vi "Data Access Client.vi"() -> ()   [LabVIEW 2019, in "OPC UA Demo.lvlib"]
doc: "Demonstrates the use of the <B>OPC UA Data Access Client VIs</B> to programmatically create an OPC UA client and connects the OPC UA client to an OPC UA server."
uses:
  OPC UA Demo.lvlib
  <vilib>/OPCUA/controls/NodeIds.ctl
  <vilib>/OPCUA/controls/NodeId.ctl
  <vilib>/OPCUA/controls/Write Variant Request.ctl
  <vilib>/OPCUA/controls/Write Status.ctl
  <vilib>/OPCUA/client/Multiple Write Variant.vi
  <vilib>/OPCUA/NI OPC UA Client.lvlib
panel:
  out "data 2":bool
  in  "stop 2":bool
  in  "security policy":T1={"message mode"=enum."Sign", "security"=enum."Basic256"}
  in  "Device.Node.Set Point":i32=1000
  out "Waveform Chart":i32(graph)
  in  "stop":bool
  in  "server endpoint URL":string="opc.tcp://localhost:49580"
  # "Overview: Demonstrates the use of the OPC UA Data Access Client VIs to programmatically create an OPC UA client and connect \nthe OPC UA client to an OPC UA server.\nRequirements: \n1. LabVIEW OPC UA Toolkit\n2. Run this VI on RT targets or Windows\nInstructions:\n1. Specify the server endpoint URL generated by the server.\n2. Specify the security policy.\n3. Run the VI."
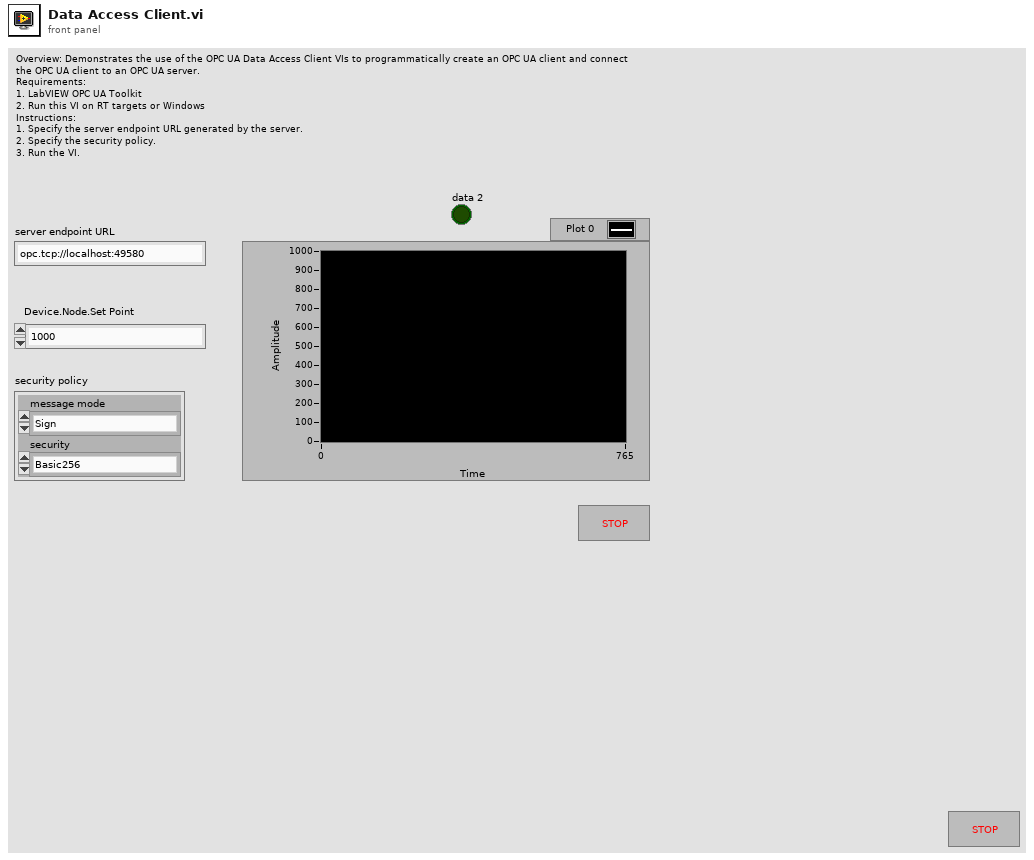
[diagram p1: front panel]
types:
  T1 = cluster{"message mode":enum16{"None", "Sign", "Sign and Encrypt"}, "security":enum16{"Basic256", "Basic128Rsa15"}}
  T2 = typedef "NodeIds.ctl" = T3[]
  T3 = typedef "NodeId.ctl" = string
  T4 = typedef "OPC UA Client Refnum.ctl" = refnum<k21>
  T5 = typedef "Subscription ID.ctl" = u32
  T6 = typedef "Subscription Data Change.ctl" = cluster{"node ID":T3, " value":variant, "timestamp":timestamp, "data type":T7, "status code":T8}
  T7 = typedef "Data Type.ctl" = u16
  T8 = typedef "OPC UA StatusCode.ctl" = u32
  T9 = typedef "Write Variant Request.ctl" = cluster{"node ID":T3, "value":variant, "timestamp (current time)":timestamp, "node status":T10}
  T10 = typedef "Write Status.ctl" = u32
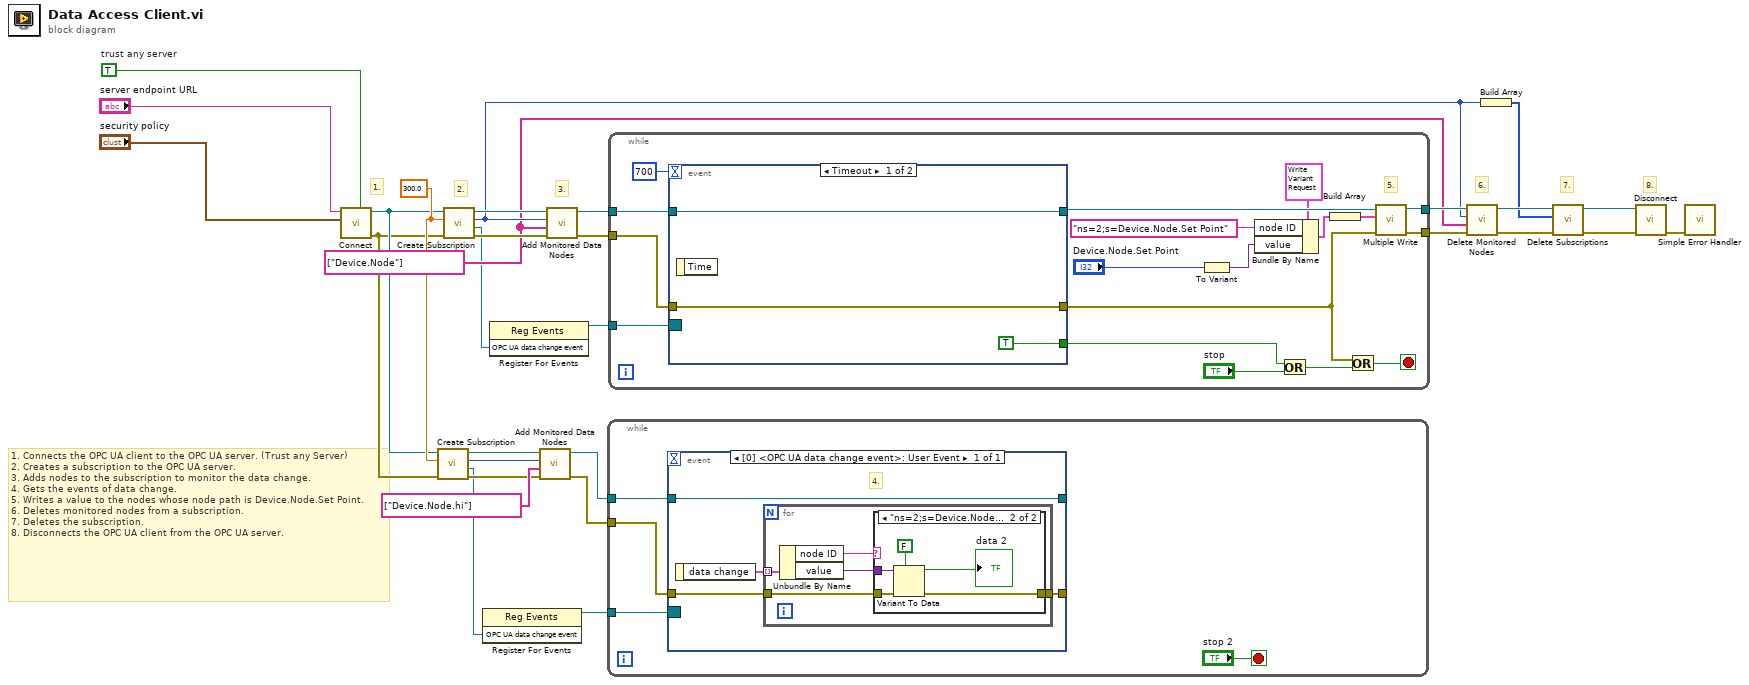
[diagram p0: block diagram]
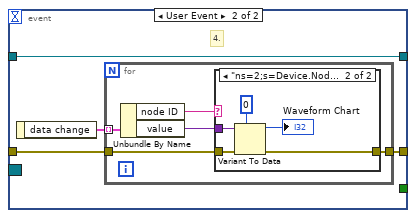
[diagram p3: hidden frame]
diagram:
  w16 = TRUE  # trust any server
  w17 = T2 ["Device.Node"] ("node IDs")
  w12 = 300.0 ("update rate (1000 ms)")
  # "7."
  # "1. Connects the OPC UA client to the OPC UA server. (Trust any Server) \n2. Creates a subscription to the OPC UA server.\n3. Adds nodes to the subscription to monitor the data change.\n4. Gets the events of data change.\n5. Writes a value to the nodes whose node path is Device.Node.Set Point. \n6. Deletes monitored nodes from a subscription.\n7. Deletes the subscription.\n8. Disconnects the OPC UA client from the OPC UA server."
  # "8."
  # "6."
  # "3."
  # "2."
  # "1."
  n1 = call <vilib>:"Connect.vi"("trust any server (F)"=w16, "security policy"="security policy", "server endpoint URL"="server endpoint URL") -> ("error out"=w7:errorcluster, "OPC UA client refnum out"=w11:T4)  [unwired: 6 in, 1 out]
  n2 = call <vilib>:"Create Subscription.vi"("error in (no error)"=w7, "publishing interval (1000 ms)"=w12, "OPC UA client refnum in"=w11) -> ("error out"=w8:errorcluster, "OPC UA data change event"=w3:refnum<user-event>, "subscription ID out"=w1:T5, "OPC UA client refnum out"=w9:T4)  [unwired: 4 in, 1 out]
  n3 = call <vilib>:"Create Subscription.vi"("error in (no error)"=w7, "publishing interval (1000 ms)"=w12, "OPC UA client refnum in"=w11) -> ("error out"=w28:errorcluster, "OPC UA data change event"=w15:refnum<user-event>, "subscription ID out"=w21:T5, "OPC UA client refnum out"=w29:T4)  [unwired: 4 in, 1 out]
  n4 = register-events(w3) -> (reference out=w2:refnum<event-registration>)  [unwired: 2 in, 1 out]
  n5 = register-events(w15) -> (reference out=w13:refnum<event-registration>)  [unwired: 2 in, 1 out]
  n6 = call <vilib>:"Add Monitored Data Nodes.vi"("error in (no error)"=w8, "node IDs"=T2 ["Device.Node.hi"], "subscription ID in"=w1, "OPC UA client refnum in"=w9) -> ("error out"=w6:errorcluster, "OPC UA client refnum out"=w4:T4)  [unwired: 4 in, 2 out]
  n7 = call <vilib>:"Add Monitored Data Nodes.vi"("error in (no error)"=w28, "node IDs"=w17, "subscription ID in"=w21, "OPC UA client refnum in"=w29) -> ("error out"=w5:errorcluster, "OPC UA client refnum out"=w14:T4)  [unwired: 4 in, 2 out]
  n8 = while {
    tunnel: w2 -> [w34]
    tunnel: w4 -> [w33]
    tunnel: w6 -> [w32]
    stop <- "stop 2" stop-if-true
    n9 = event shown="[0] <OPC UA data change event>: User Event" {
      selector: w34 -> [_]
      dyn-events: _ -> [_]
      timeout: _ -> [_]
      tunnel: w33 -> [w35]
      tunnel: [w35] -> _
      tunnel: [w36] -> _
      tunnel: w32 -> [w37]
      event User Event {
        # "4."
        n10 = event-data() -> ("data change"=w38:T6[])  [unwired: 1 in]
        n11 = for {
          tunnel: w38 -> [w40] mode=indexing
          tunnel: w37 -> [w42]
          tunnel: [w41] -> w36
          n12 = Unbundle By Name(w40) -> ("node ID"=w39:T3, "value"=w43:variant)
          n13 = case shown="\"ns=2;s=Device.Node.hi\"" w39 {
            tunnel: w43 -> [_ w49]
            tunnel: w42 -> [w44 w47]
            tunnel: [w44 w46] -> w41
            frame "False", Default {
            }
            frame "ns=2;s=Device.Node.hi" {
              n14 = Variant To Data(error in=w47, type=FALSE, Variant=w49) -> (data=→"data 2":bool, error out=w46:errorcluster)
            }
          }
        }
      }
    }
  }
  n15 = while {
    tunnel: w13 -> [w67]
    tunnel: w14 -> [w65]
    tunnel: w5 -> [w61]
    tunnel: [w62] -> w26
    tunnel: [w63] -> w27
    stop <- w54 stop-if-true
    # "5."
    n16 = event shown="[0] Timeout" {
      selector: w67 -> [_ _]
      dyn-events: _ -> [_ _]
      timeout: 700 -> [_ _]
      tunnel: w65 -> [w70 w71]
      tunnel: [w70 w71] -> w64
      tunnel: [w69 w72] -> w53
      tunnel: w61 -> [w69 w73]
      tunnel: [TRUE _] -> w51
      event Timeout {
        n17 = event-data() -> ()  [unwired: 1 in, 1 out]
      }
      event User Event {
        # "4."
        n18 = event-data() -> ("data change"=w74:T6[])  [unwired: 1 in]
        n19 = for {
          tunnel: w74 -> [w76] mode=indexing
          tunnel: w73 -> [w78]
          tunnel: [w77] -> w72
          n20 = Unbundle By Name(w76) -> ("node ID"=w75:T3, "value"=w79:variant)
          n21 = case shown="\"ns=2;s=Device.Node\"" w75 {
            tunnel: w79 -> [_ w85]
            tunnel: w78 -> [w80 w82]
            tunnel: [w80 w81] -> w77
            frame "False", Default {
            }
            frame "ns=2;s=Device.Node" {
              n22 = Variant To Data(error in=w82, type=0, Variant=w85) -> (data=→"Waveform Chart":i32, error out=w81:errorcluster)
            }
          }
        }
      }
    }
    n23 = To Variant(anything="Device.Node.Set Point") -> (Variant=w59:variant)
    n24 = Bundle By Name(cluster=T9 {"node ID"="", "value"=variant, "timestamp (current time)"=timestamp(0 s since 1904-01-01), "node status"=0} ("request"), "node ID"=T3 "ns=2;s=Device.Node.Set Point", "value"=w59) -> (w56:T9)
    n25 = Or(x=w51, y="stop") -> (x .or. y?=w50:bool)
    n26 = Build Array(w56) -> (w55:T9[])
    n27 = Or(x=w53, y=w50) -> (x .or. y?=w54:bool)
    n28 = call-poly <vilib>:"Multiple Write.vi"("error in (no error)"=w53, "requests"=w55, "OPC UA client refnum in"=w64) -> ("error out"=w62:errorcluster, "OPC UA client refnum out"=w63:T4)  [unwired: 5 in, 2 out]
  }
  n29 = call <vilib>:"Delete Monitored Nodes.vi"("error in (no error)"=w26, "node IDs"=w17, "subscription ID in"=w21, "OPC UA client refnum in"=w27) -> ("error out"=w24:errorcluster, "OPC UA client refnum out"=w25:T4)  [unwired: 3 in, 3 out]
  n30 = Build Array(w21) -> (w20:T5[])
  n31 = call <vilib>:"Delete Subscriptions.vi"("error in (no error)"=w24, "subscription IDs"=w20, "OPC UA client refnum in"=w25) -> ("error out"=w22:errorcluster, "OPC UA client refnum out"=w23:T4)  [unwired: 6 in, 1 out]
  n32 = call <vilib>:"Disconnect.vi"("error in (no error)"=w22, "OPC UA client refnum in"=w23) -> ("error out"=w18:errorcluster)  [unwired: 9 in]
  n33 = call <vilib>:"Simple Error Handler.vi"("error in (no error)"=w18) -> ()  [unwired: 4 in, 5 out]
